vi "setRampParameters.vi"(8 "error in (no error)":errorcluster, 10 "RampParameters":T1, 11 "RampEvent in":refnum<class "RampEvent.lvclass">) -> (0 "error out":errorcluster, 3 "RampEvent out":refnum<class "RampEvent.lvclass">)   [LabVIEW 2009, in "Tools.lvlib" / "Scripting.lvlib" / "RampEvent.lvclass"]
uses:
  RampEvent.lvclass
  RampEvent.lvclass/RampEvent.ctl
  ScriptEvent.lvclass
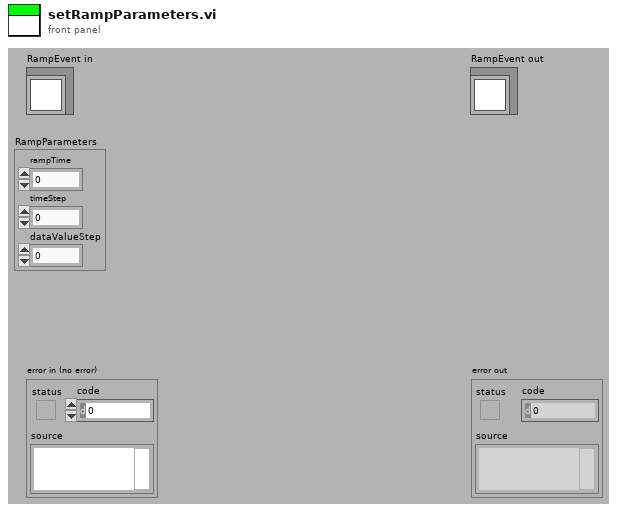
[diagram p1: front panel]
types:
  T1 = cluster{"rampTime":dbl, "timeStep":dbl, "dataValueStep":dbl}
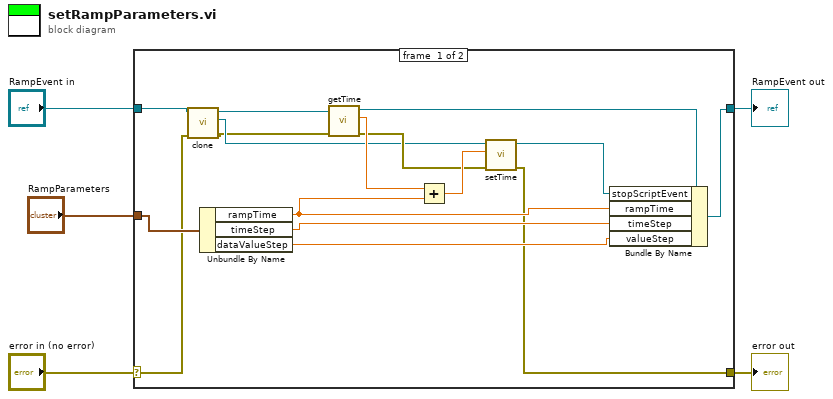
[diagram p0: block diagram]
diagram:
  n1 = case shown="No Error" "error in (no error)" {
    selector: "error in (no error)" -> [w13 w23]
    tunnel: [w7 w23] -> w4
    tunnel: [w8 w22] -> w2
    tunnel: "RampEvent in" -> [w16 w22]
    tunnel: "RampParameters" -> [w21 _]
    frame #0 {
      n2 = call-dynamic "clone.vi"("error in (no error)"=w13, "ScriptEvent in"=w16) -> ("error out"=w14:errorcluster, "clone"=w17:refnum<class "ScriptEvent.lvclass">, "ScriptEvent out"=w15:refnum<class "RampEvent.lvclass">)  [unwired: 7 in]
      n3 = Unbundle By Name(w21) -> ("rampTime"=w12:dbl, "timeStep"=w11:dbl, "dataValueStep"=w10:dbl)
      n4 = call "getTime.vi"("error in (no error)"=w14, "ScriptEvent.lvclass in"=w15) -> ("error out"=w18:errorcluster, "time"=w20:dbl, "ScriptEvent.lvclass out"=w9:refnum<class "RampEvent.lvclass">)  [unwired: 7 in]
      n5 = Add(x=w20, y=w12) -> (x+y=w19:dbl)
      n6 = call "setTime.vi"("error in (no error)"=w18, "time"=w19, "ScriptEvent.lvclass in"=w17) -> ("error out"=w7:errorcluster, "ScriptEvent.lvclass out"=w6:refnum<class "ScriptEvent.lvclass">)  [unwired: 7 in]
      n7 = Bundle By Name(cluster=w9, "stopScriptEvent"=w6, "rampTime"=w12, "timeStep"=w11, "valueStep"=w10) -> (w8:refnum<class "RampEvent.lvclass">)
    }
    frame #1 {
    }
  }
  "error out" <- w4
  "RampEvent out" <- w2
